vi "Register Sessions.vi"(8 "error in (no error)":errorcluster, 10 "data in":T1, 11 "state in":refnum<class "Unreserved State.lvclass">) -> (0 "error out":errorcluster, 2 "data out":T1)   [LabVIEW 2020, in "MeasurementLink Session Management.lvlib" / "Unreserved State.lvclass"]
uses:
  Unreserved State.lvclass
  MeasurementLink Measurement Server/Helpers/Error Strings Global Internal.vi
  IState/IState.lvclass
  MeasurementLink Session Management Client/RPC Messages/ni_measurementlink_sessionmanagement_v1_ChannelMapping.ctl
  MeasurementLink Session Management Client/MeasurementLink Session Management Client.lvlib
  MeasurementLink Session Management Client/RPC Messages/nidevice_grpc_Session.ctl
  MeasurementLink Session Management Client/RPC Messages/ni_measurementlink_sessionmanagement_v1_SessionInformation.ctl
  MeasurementLink Instrument/IInstrument/IInstrument.lvclass
  Session Reservation/Session and Driver Info.ctl
  Session Reservation/Session Reservation.lvclass
  MeasurementLink Session Management Client/RPC Messages/ni_measurementlink_PinMapContext.ctl
  Connection Map/Connection Map.lvclass
  Session Reservation/Data.ctl
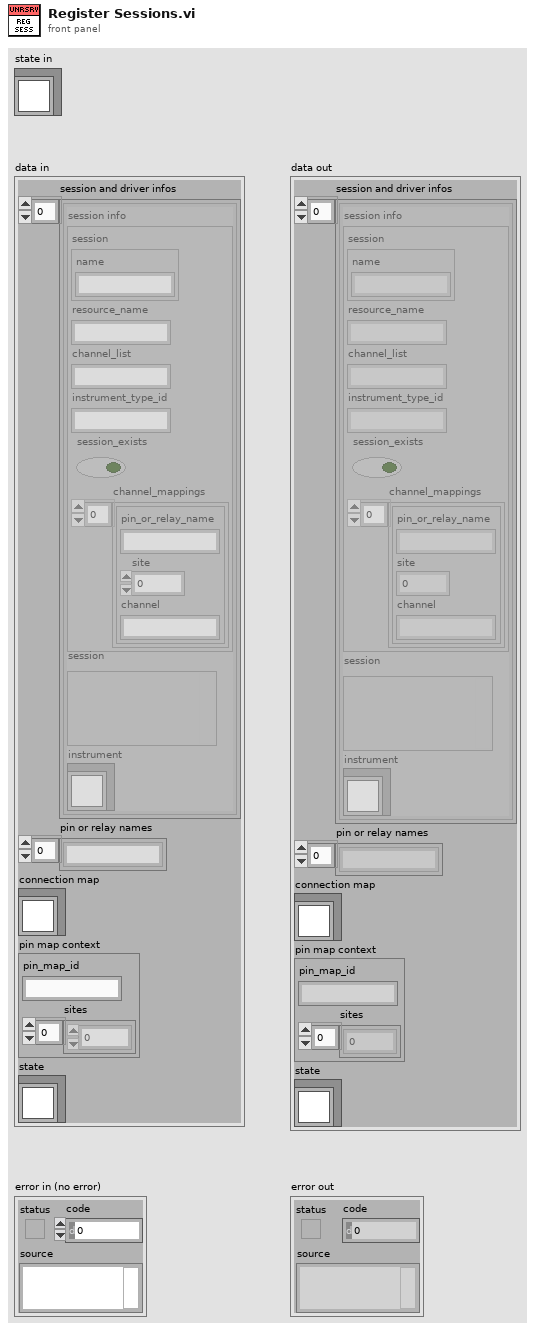
[diagram p1: front panel]
types:
  T1 = typedef "MeasurementLink Session Management.lvlib/Session Reservation.lvclass/Data.ctl" = cluster{"session and driver infos":T2[], "pin or relay names":string[], "connection map":refnum<class "Connection Map.lvclass">, "pin map context":T6, "state":refnum<class "IState.lvclass">}
  T2 = typedef "MeasurementLink Session Management.lvlib/Session Reservation.lvclass/Session and Driver Info.ctl" = cluster{"session info":T3, "session":variant, "instrument":refnum<class "IInstrument.lvclass">}
  T3 = typedef "MeasurementLink Session Management Client.lvlib/ni_measurementlink_sessionmanagement_v1_SessionInformation.ctl" = cluster{"session":T4, "resource_name":string, "channel_list":string, "instrument_type_id":string, "session_exists":bool, "channel_mappings":T5[]}
  T4 = typedef "MeasurementLink Session Management Client.lvlib/nidevice_grpc_Session.ctl" = cluster{"name":string}
  T5 = typedef "MeasurementLink Session Management Client.lvlib/ni_measurementlink_sessionmanagement_v1_ChannelMapping.ctl" = cluster{"pin_or_relay_name":string, "site":i32, "channel":string}
  T6 = typedef "MeasurementLink Session Management Client.lvlib/ni_measurementlink_PinMapContext.ctl" = cluster{"pin_map_id":string, "sites":i32[]}
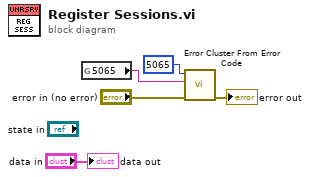
[diagram p0: block diagram]
diagram:
  n1 = global read "Error Strings Global Internal.vi" "5065"() -> (w5:string)
  n2 = call <vilib>:"Error Cluster From Error Code.vi"("error in (no error)"="error in (no error)", "error message (\"\")"=w5, "error code (0)"=5065) -> ("error out"=→"error out":errorcluster)  [unwired: 6 in]
  "data out" <- "data in"
